vi "PRIME Detector Read All Responses.vi"(7 "Log":bool, 8 "error in":errorcluster, 10 "Str Ref":refnum<vi>, 11 "connection ID":refnum<k5>) -> (0 "error out":errorcluster, 1 "Responses":string[](array[string]), 2 "Status Response":string, 3 "connection ID out":refnum<k5>)   [LabVIEW 2024, in "PRIME Detector.lvclass"]
uses:
  PRIME Detector.lvclass
  <vilib>/Utility/error.llb/Trim Whitespace One-Sided.vi
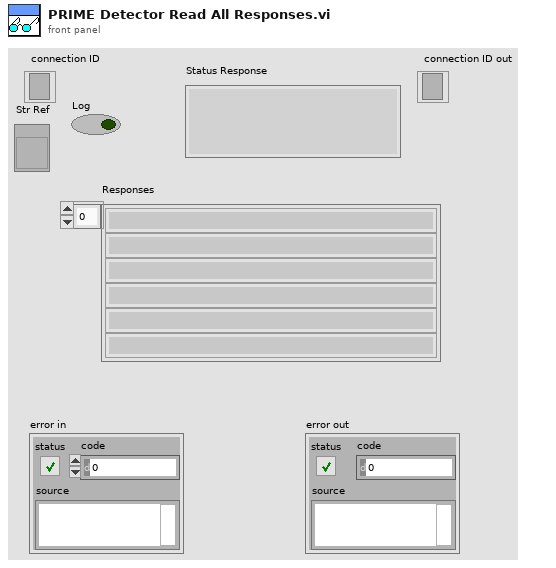
[diagram p1: front panel]
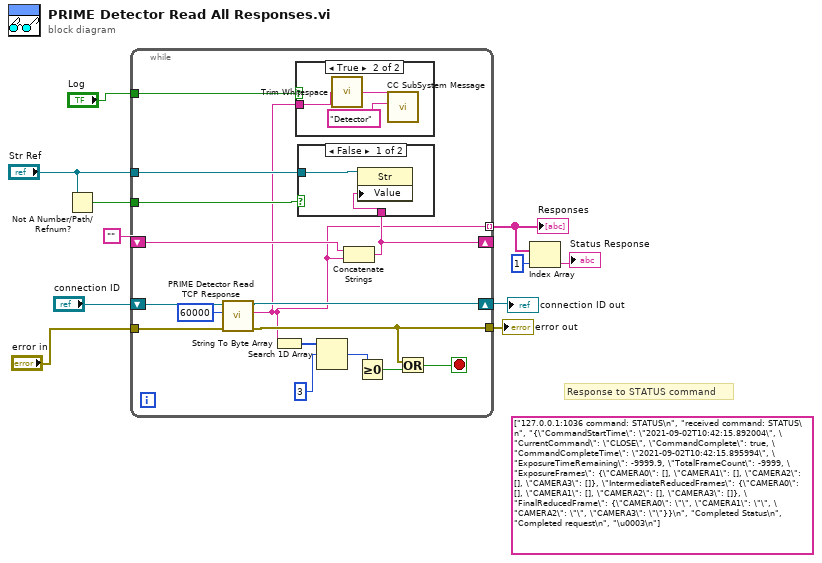
[diagram p0: block diagram]
diagram:
  (unwired) string[] ["127.0.0.1:1036 command: STATUS\n", "received command: STATUS\n", "{\"CommandStartTime\": \"2021-09-02T10:42:15.892004\", \"CurrentCommand\": \"CLOSE\", \"CommandComplete\": true, \"CommandCompleteTime\": \"2021-09-02T10:42:15.895994\", \"ExposureTimeRemaining\": -9999.9, \"TotalFrameCount\": -9999, \"ExposureFrames\": {\"CAMERA0\": [], \"CAMERA1\": [], \"CAMERA2\": [], \"CAMERA3\": []}, \"IntermediateReducedFrames\": {\"CAMERA0\": [], \"CAMERA1\": [], \"CAMERA2\": [], \"CAMERA3\": []}, \"FinalReducedFrame\": {\"CAMERA0\": \"\", \"CAMERA1\": \"\", \"CAMERA2\": \"\", \"CAMERA3\": \"\"}}\n", "Completed Status\n", "Completed request\n", "\u0003\n"] ("Responses")
  # "Response to STATUS command"
  n1 = Not A Number/Path/Refnum?(number/path/refnum="Str Ref") -> (NaN/Path/Refnum?=w4:bool)
  n2 = while {
    tunnel: "error in" -> [w26]
    tunnel: [w21] -> w7
    tunnel: [w12] -> w11 mode=indexing
    shift-right: [w25] -> w5
    shift-left: "connection ID" -> [w27]
    tunnel: w4 -> [w17]
    tunnel: "Str Ref" -> [w16]
    shift-right: [w14] -> _
    shift-left: "" -> [w15]
    tunnel: "Log" -> [w13]
    stop <- w22 stop-if-true
    n3 = call "PRIME Detector Read TCP Response.vi"("error in (no error)"=w26, "timeout ms (6000)"=60000, "connection ID"=w27) -> ("error out"=w21:errorcluster, "response message"=w12:string, "connection ID out"=w25:refnum<k5>)  [unwired: 5 in, 1 out]
    n4 = String To Byte Array(string=w12) -> (unsigned byte array=w20:u8[])
    n5 = case shown="True" w13 {
      tunnel: w12 -> [_ w30]
      frame False {
      }
      frame True {
        n6 = call <vilib>:"Trim Whitespace.vi"("string"=w30) -> ("trimmed string"=w29:string)  [unwired: 1 in]
        n7 = call "CC SubSystem Message.vi"("Subsystem"="Detector", "Message"=w29) -> ()  [unwired: 9 in, 1 out]
      }
    }
    n8 = Search 1D Array(1D array=w20, element=u8 3 ("y")) -> (index of element=w24:i32)  [unwired: 1 in]
    n9 = Concatenate Strings(w15, w12) -> (w14:string)
    n10 = case shown="False" w17 {
      tunnel: w16 -> [w32 _]
      tunnel: w14 -> [w31 _]
      frame False {
        n11 = property class="Str"(reference=w32, "Value"=w31) -> ()  [unwired: 1 in, 2 out]
      }
      frame True {
      }
    }
    n12 = Greater Or Equal To 0?(x=w24) -> (x >= 0?=w23:bool)
    n13 = Or(x=w21, y=w23) -> (x .or. y?=w22:bool)
  }
  "Responses" <- w11
  "error out" <- w7
  "connection ID out" <- w5
  n14 = Index Array(array=w11, index=1) -> (element=→"Status Response":string)
